vi "Task Done.vi"(8 "error in (no error)":errorcluster, 11 "NI PWM Input in":refnum<class "NI PWM Input.lvclass">) -> (0 "error out":errorcluster, 3 "NI PWM Input out":refnum<class "NI PWM Input.lvclass">)   [LabVIEW 2023, in "HardwareAbstractionLayer_LVOOP.lvlib" / "NI PWM Input.lvclass"]
uses:
  NI PWM Input.lvclass
  NI PWM Input.lvclass/NI PWM Input.ctl
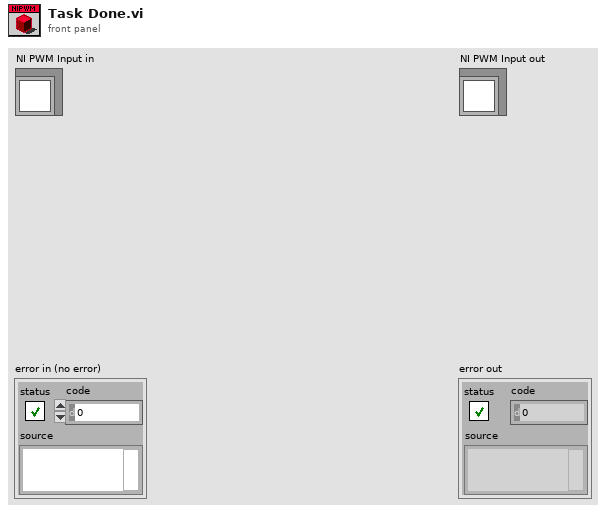
[diagram p1: front panel]
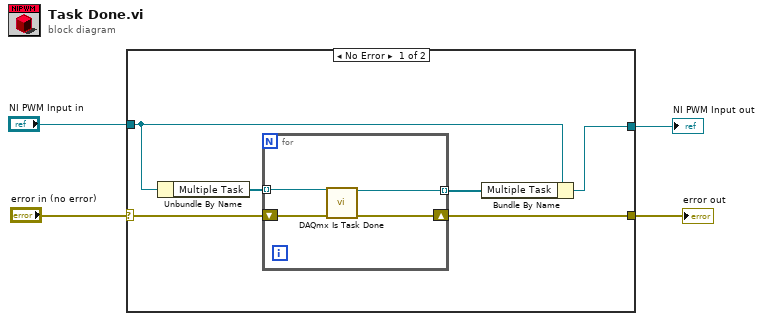
[diagram p0: block diagram]
diagram:
  n1 = case shown="No Error" "error in (no error)" {
    selector: "error in (no error)" -> [w9 w15]
    tunnel: "NI PWM Input in" -> [w7 w16]
    tunnel: [w8 w15] -> w2
    tunnel: [w5 w16] -> w1
    frame No Error {
      n2 = Unbundle By Name(w7) -> ("Multiple Task"=w10:refnum<k21>[])
      n3 = for {
        tunnel: w10 -> [w14] mode=indexing
        tunnel: [w13] -> w6 mode=indexing
        shift-right: [w11] -> w8
        shift-left: w9 -> [w12]
        n4 = call <vilib>:"DAQmx Is Task Done.vi"("task/channels in"=w14, "error in"=w12) -> ("task out"=w13:refnum<k21>, "error out"=w11:errorcluster)  [unwired: 11 in, 1 out]
      }
      n5 = Bundle By Name(cluster=w7, "Multiple Task"=w6) -> (w5:refnum<class "NI PWM Input.lvclass">)
    }
    frame Error {
    }
  }
  "error out" <- w2
  "NI PWM Input out" <- w1
